vi "RegisterDataSetsRoutedMessage_Send.vi"(8 "error in (no error)":errorcluster, 10 "RegisterDataSet":T1, 11 "Qbus in":refnum<class "Qbus.lvclass">) -> (0 "error out":errorcluster, 3 "Qbus out":refnum<class "Qbus.lvclass">)   [LabVIEW 2017, in "McsaDataEventCreator.lvlib"]
doc: "Provides the TDMS Creator process with information about trends calculated from channel data. Trends must be registered with TDMS Creator, otherwise the TDMS Creator process does not write their values to file."
uses:
  <vilib>/addons/InsightCM/Devices/Shared/Mcsa/McsaDataEventCreator/McsaDataEventCreator.lvlib
  <vilib>/addons/Qbus/Qbus.lvclass
  <vilib>/addons/InsightCM/Devices/Shared/Mcsa/McsaDataEventCreator/controls/RegisterDataSets.ctl
  <vilib>/addons/InsightCM/Devices/Shared/Mcsa/McsaDataEventCreator/controls/Registry_DataSet.ctl
  <vilib>/addons/InsightCM/Devices/Shared/Mcsa/McsaDataEventCreator/controls/DataSetType.ctl
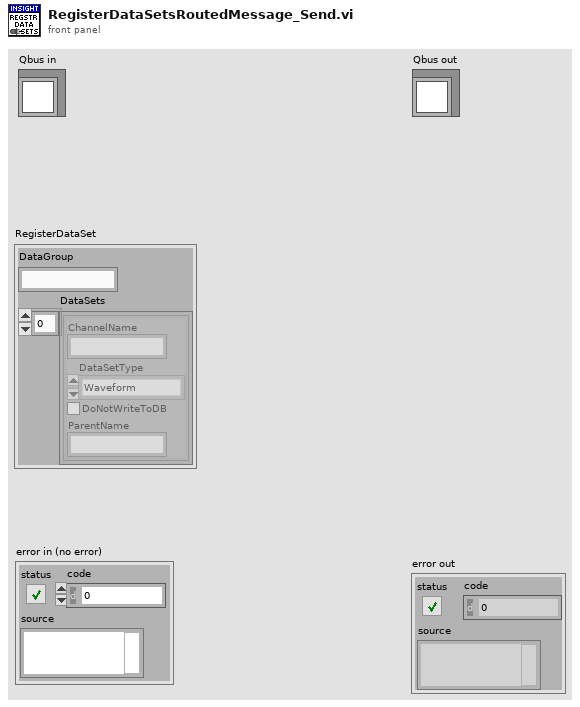
[diagram p1: front panel]
types:
  T1 = typedef "McsaDataEventCreator.lvlib/RegisterDataSets.ctl" = cluster{"DataGroup":string, "DataSets":T2[]}
  T2 = typedef "McsaDataEventCreator.lvlib/Registry_DataSet.ctl" = cluster{"ChannelName":string, "DataSetType":T3, "DoNotWriteToDB":bool, "ParentName":string}
  T3 = typedef "McsaDataEventCreator.lvlib/DataSetType.ctl" = enum16{"Waveform", "MCSAFFT", "TorqueWFM"}
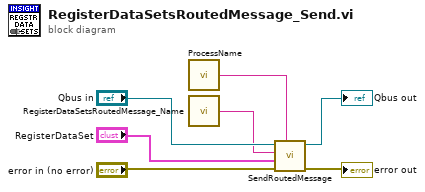
[diagram p0: block diagram]
diagram:
  n1 = call <vilib>:"ProcessName.vi"() -> ("process name"=w2:string)  [unwired: 5 in]
  n2 = call <vilib>:"RegisterDataSetsRoutedMessage_Name.vi"() -> ("message name"=w1:string)  [unwired: 5 in]
  n3 = call <vilib>:"SendRoutedMessage.vi"("listener process"=w2, "error in (no error)"="error in (no error)", "message value"="RegisterDataSet", "message name"=w1, "Qbus in"="Qbus in") -> ("error in (no error)"=→"error out":errorcluster, "Qbus out"=→"Qbus out":refnum<class "Qbus.lvclass">)  [unwired: 5 in]
